vi "StripTimeFromTimeStamp.vi"(4 "current time":timestamp) -> (1 "date only":timestamp)   [LabVIEW 2024]
uses:
  <vilib>/Utility/miscctls.llb/LVDateTimeRec.ctl
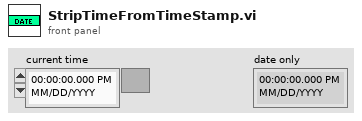
[diagram p1: front panel]
types:
  T1 = typedef "LVDateTimeRec.ctl" = cluster{"fractional second":dbl, "second":i32, "minute":i32, "hour":i32, "day of month":i32, "month":i32, "year":i32, "day of week":i32, "day of year":i32, "DST":i32}
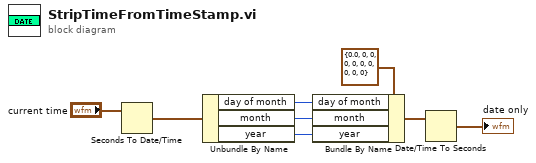
[diagram p0: block diagram]
diagram:
  n1 = Seconds To Date/Time(time stamp (now)="current time") -> (date time rec=w7:T1)  [unwired: 1 in]
  n2 = Unbundle By Name(w7) -> ("day of month"=w4:i32, "month"=w3:i32, "year"=w2:i32)
  n3 = Bundle By Name(cluster=T1 {"fractional second"=0.0, "second"=0, "minute"=0, "hour"=0, "day of month"=0, "month"=0, "year"=0, "day of week"=0, "day of year"=0, "DST"=0} ("date time rec"), "day of month"=w4, "month"=w3, "year"=w2) -> (w5:T1)
  n4 = Date/Time To Seconds(2:w5) -> (0:→"date only":timestamp)  [unwired: 1 in]
